vi "spec_set_cupconfig.vi"(8 "error in (no error)":errorcluster, 9 "supcub config name":string, 10 "cup config name":string, 11 "Qtegra in":refnum<class "Qtegra.lvclass">) -> (0 "error out":errorcluster, 2 "value out":string, 3 "Qtegra out":refnum<class "Qtegra.lvclass">)   [LabVIEW 2018, in "Qtegra.lvclass"]
doc: "set the cup and subcup configuration of the instrument\n\nmainly for qtegra"
uses:
  Qtegra.lvclass
  \\Mac\Home/my data/privat/Software/LabView/MSControlSuite_Code/MSControl/Classes/Instrument/instrument.lvclass
  global variables.vi
  instrument.lvclass
  StatusLog/StatusLog.lvclass
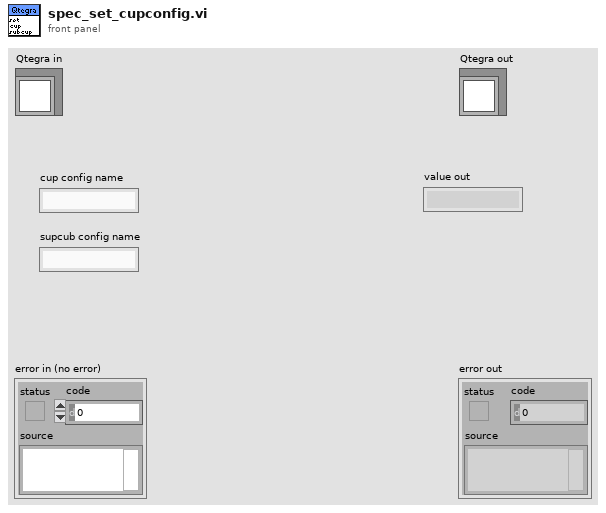
[diagram p1: front panel]
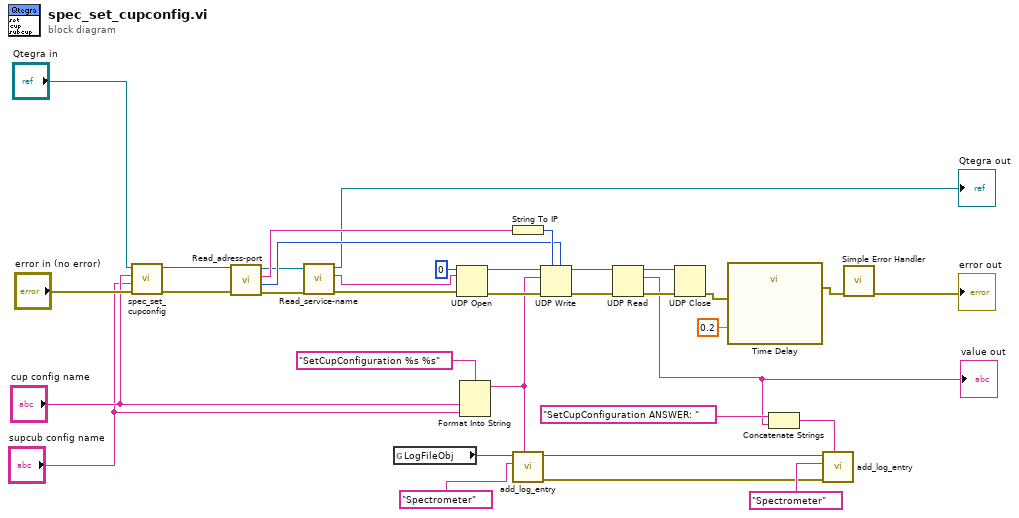
[diagram p0: block diagram]
diagram:
  n1 = call-parent "spec_set_cupconfig.vi"("error in (no error)"="error in (no error)", "supcub config name"="supcub config name", "cup config name"="cup config name", "instrument in"="Qtegra in") -> ("error out"=w6:errorcluster, "instrument out"=w7:refnum<class "Qtegra.lvclass">)  [unwired: 5 in, 1 out]
  n2 = call "Read_adress-port.vi"("error in (no error)"=w6, "instrument in"=w7) -> ("error out"=w25:errorcluster, "port number"=w26:i32, "adress"=w33:string, "instrument out"=w24:refnum<class "Qtegra.lvclass">)  [unwired: 6 in]
  n3 = call-dynamic "Read_service-name.vi"("error in (no error)"=w25, "instrument in"=w24) -> ("error out"=w23:errorcluster, "service name"=w22:string, "instrument out"=→"Qtegra out":refnum<class "Qtegra.lvclass">)  [unwired: 7 in]
  n4 = global read "global variables.vi" "LogFileObj"() -> (w12:refnum<class "StatusLog.lvclass">)
  n5 = UDP Open(8:w23, 10:w22, 11:u16 0 ("port")) -> (port=w29:refnum<k16>, 0:w30:errorcluster)  [unwired: 2 in, 1 out]
  n6 = Format Into String(format string="SetCupConfiguration %s %s", "cup config name", "supcub config name") -> (resulting string=w14:string)  [unwired: 2 in, 1 out]
  n7 = String To IP(1:w33) -> (0:w32:u32)
  n8 = call-dynamic "add_log_entry.vi"("new entry"=w14, "log identifiers"="Spectrometer", "StatusLog in"=w12) -> ("error out"=w8:errorcluster, "StatusLog out"=w11:refnum<class "StatusLog.lvclass">)  [unwired: 5 in]
  n9 = UDP Write(address=w32, port or service name=w26, connection ID=w29, data in=w14, 8:w30) -> (error out=w27:errorcluster, 3:w28:refnum<k16>)  [unwired: 1 in]
  n10 = UDP Read(connection ID=w28, 8:w27) -> (data out=w2:string, error out=w20:errorcluster, 3:w19:refnum<k16>)  [unwired: 2 in, 2 out]
  "value out" <- w2
  n11 = UDP Close(connection ID=w19, 8:w20) -> (error out=w18:errorcluster)  [unwired: 1 out]
  n12 = call "Time Delay"("error in (no error)"=w18, "Delay Time (s)"=0.2) -> ("error out"=w17:errorcluster)  [unwired: 9 in]
  n13 = Concatenate Strings("SetCupConfiguration ANSWER: ", w2) -> (w9:string)
  n14 = call-dynamic "add_log_entry.vi"("new entry"=w9, "error in (no error)"=w8, "log identifiers"="Spectrometer", "StatusLog in"=w11) -> ()  [unwired: 4 in, 2 out]
  n15 = call <vilib>:"Simple Error Handler.vi"("error in (no error)"=w17) -> ("error out"=→"error out":errorcluster)  [unwired: 4 in, 4 out]
